vi "Periodic Tasks.vi"(8 "error in (no error)":errorcluster) -> ()   [LabVIEW 2015]
doc: "This VI runs in parallel to other tasks. It can contain as many user-defined periodic loops as you need. These can carry out PID or other sorts of timed response."
uses:
  <vilib>/Rock Robotics/WPI/DriverStation/WPI_DriverStationRobotMode2.ctl
  <vilib>/Rock Robotics/WPI/CAN/TalonSRX/WPI_CANTalonSRX_APIControlMode.ctl
  <vilib>/Rock Robotics/WPI/Utilities/WPI_GetSetVariantRefNum.vi
  Robot Global Data.vi
  <vilib>/Rock Robotics/Network Tables/NT Write Number.vi
  <vilib>/Rock Robotics/Network Tables/NT Write Boolean.vi
  <vilib>/Rock Robotics/Network Tables/SD Read Boolean.vi
  <vilib>/Rock Robotics/Network Tables/SD Write Number.vi
  navX-MXP-LabVIEW/navX-MXP Library/navX-MXP IMU.lvlib
  <vilib>/Rock Robotics/WPI/DriverStation/WPI_DriverStationAllianceInfo.ctl
  900/Team900-VIs/Team900SwerveDrive/Team900SwerveDrive.lvlib
  <vilib>/Rock Robotics/Network Tables/SD Read Number.vi
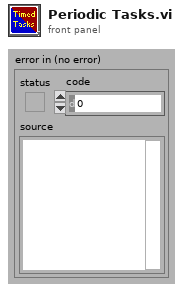
[diagram p1: front panel]
types:
  T1 = typedef "WPI_DriverStationRobotMode2.ctl" = enum16{"Autonomous Disabled", "Autonomous Enabled", "Teleop Disabled", "Teleop Enabled", "Disconnected", "Finish", "Test Disabled", "Test Enabled", "Emergency Stopped"}
  T2 = typedef "WPI_CANTalonSRX_APIControlMode.ctl" = enum8{"Percent VBus", "Speed", "Position", "Slave", "Unchanged / Invalid"}
  T3 = typedef "WPI_MotorControlDeviceRef.ctl" = cluster{"DeviceStatus":errorcluster, "Type":T4, "PWM":cluster{"PWM Channel":T5, "DeadBand":T6}, "CAN":cluster{"Device Number":u8, "Control Mode":T7, "Semaphore":T8, "Max Vout":dbl, "TalonSRX Control Mode":T2}, "Invert":bool, "TransformRef":T9, "InvTransformRef":T9}
  T4 = typedef "WPI_MotorControlType.ctl" = enum16{"PWM", "CAN", "CANTalonSRX"}
  T5 = typedef "FPGA_DIOPWMChannel.ctl" = enum8{"PWM 0", "PWM 1", "PWM 2", "PWM 3", "PWM 4", "PWM 5", "PWM 6", "PWM 7", "PWM 8", "PWM 9", "PWM MXP 0", "PWM MXP 1", "PWM MXP 2", "PWM MXP 3", "PWM MXP 4", "PWM MXP 5", "PWM MXP 6", "PWM MXP 7", "PWM MXP 8", "PWM MXP 9", "Invalid"}
  T6 = typedef "WPI_PWMDeadband.ctl" = cluster{"Name":string, "maxPositivePwm":i32, "minPositivePwm":i32, "centerPwm":i32, "maxNegativePwm":i32, "minNegativePwm":i32, "angularRange":u16}
  T7 = typedef "WPI_CANJaguar_ControlMode.ctl" = enum8{"Percent VBus", "Current", "Speed", "Position", "Voltage"}
  T8 = typedef "Semaphore RefNum" = refnum<k1>
  T9 = typedef "WPI_PWMTransform_ConPane.ctl" = refnum<vi>
  T10 = typedef "WPI_DriverStationAllianceInfo.ctl" = enum16{"Red", "Blue", "Invalid"}
  T11 = cluster{"FL Steering":T3, "FR Steering":T3, "RL Steering":T3, "RR Steering":T3}
  T12 = cluster{"FL Speed":T3, "FR Speed":T3, "RL Speed":T3, "RR Speed":T3}
  T13 = typedef "navX-MXP IMU.lvlib/navX Device TypeDef.ctl" = cluster{"navX Interface Protocol":T14, "navX Interface Protocol TypeDefs":cluster{"SPIDevRef":T15, "I2CDevRef":T17}, "navX System Information":cluster{"Board Information":T19, "Status":T20, "Offsets":T24}, "navX Common Information":cluster{"Update Rate (4Hz-60Hz)":T25, "refnum name":string, "error":errorcluster}}
  T14 = typedef "navX-MXP IMU.lvlib/navX Interface Protocol.ctl" = enum16{"SPI", "I2C"}
  T15 = typedef "WPI_SPIDevRef.ctl" = cluster{"DevStatus":errorcluster, "Handle":i32, "SPI Bus":T16}
  T16 = typedef "spi_bus.ctl" = enum16{"SPI On-Board, CS0", "SPI On-Board, CS1", "SPI On-Board, CS2", "SPI On-Board, CS3", "SPI MXP", "Invalid"}
  T17 = typedef "WPI_I2CDevRef.ctl" = cluster{"DevStatus":errorcluster, "Device Address":u8, "Handle":i32, "I2C Bus":T18}
  T18 = typedef "i2c_bus.ctl" = enum16{"I2C On-Board", "I2C MXP", "Invalid"}
  T19 = typedef "navX-MXP IMU.lvlib/navX Board Information.ctl" = cluster{"WhoAmI (50 | 0x32)":u8, "Board Revision":u8, "Firmware Major Version":u8, "Firmware Minor Version":u8}
  T20 = typedef "navX-MXP IMU.lvlib/navX Status Data.ctl" = cluster{"Update Rate Hz":u8, "Accelerometer Full-Scale Range":u8, "Gyro Full-Scale Range":u16, "NAVX_OP_STATUS":T21, "NAVX_CAL_STATUS":T22, "NAVX_SELFTEST_STATUS":u8, "NAVX_SENSOR_STATUS":T23}
  T21 = typedef "navX-MXP IMU.lvlib/navX NAVX_OP_STATUS.ctl" = u8
  T22 = typedef "navX-MXP IMU.lvlib/navX NAVX_CAL_STATUS.ctl" = u8
  T23 = typedef "navX-MXP IMU.lvlib/navX NAVX_SENSOR_STATUS.ctl" = cluster{"MOVING":bool, "YAW_STABLE":bool, "MAG_DISTURBANCE":bool, "ALTITUDE_VALID":bool, "SEALEVEL_PRESS_SET":bool, "FUSED_HEADING_VALID":bool}
  T24 = typedef "navX-MXP IMU.lvlib/navX Offsets Data.ctl" = cluster{"Yaw":dbl, "Quat W":dbl, "Quat X":dbl, "Quat Y":dbl, "Quat Z":dbl}
  T25 = typedef "navX-MXP IMU.lvlib/navX Update Rate.ctl" = u8
  T26 = typedef "navX-MXP IMU.lvlib/navX YPRH Data.ctl" = cluster{"Yaw":dbl, "Pitch":dbl, "Roll":dbl, "Heading":dbl}
  T27 = typedef "WPI_CANTalonSRX_GlobalStatus.ctl" = cluster{"Applied Throttle":dbl, "Module Enabled":bool, "CAN Error":errorcluster, "Closed Loop Error":dbl, "Forward Limit Switch Closed":bool, "Reverse Limit Switch Closed":bool, "Sensor Position":dbl, "Sensor Velocity":dbl, "Current":dbl, "Sticky Fault - Over Temp":bool, "Sticky Fault - Under Voltage":bool, "Sticky Fault - Forward Limit":bool, "Sticky Fault - Reverse Limit":bool, "Sticky Fault - Forward Soft Limit":bool, "Sticky Fault - Reverse Soft Limit":bool, "Brake is Enabled":bool, "Encoder Position":dbl, "Encoder Velocity":dbl, "Encoder Index Count":dbl, "Encoder A Pin State":bool, "Encoder B Pin State":bool, "Encoder Index Pin State":bool, "Analog In":dbl, "Analog In Velocity":dbl, "Temperature (C)":dbl, "Battery Voltage":dbl}
  T28 = cluster{"[0]":dbl, "[1]":dbl, "[2]":dbl, "[3]":dbl}
  T29 = typedef "WPI_DriverStationPositionInfo.ctl" = enum16{"1", "2", "3"}
  T30 = typedef "WPI_JoystickDevRef.ctl" = cluster{"Device":T31}
  T31 = typedef "WPI_JoystickDeviceEnum.ctl" = enum16{"USB 0", "USB 1", "USB 2", "USB 3", "USB 4", "USB 5"}
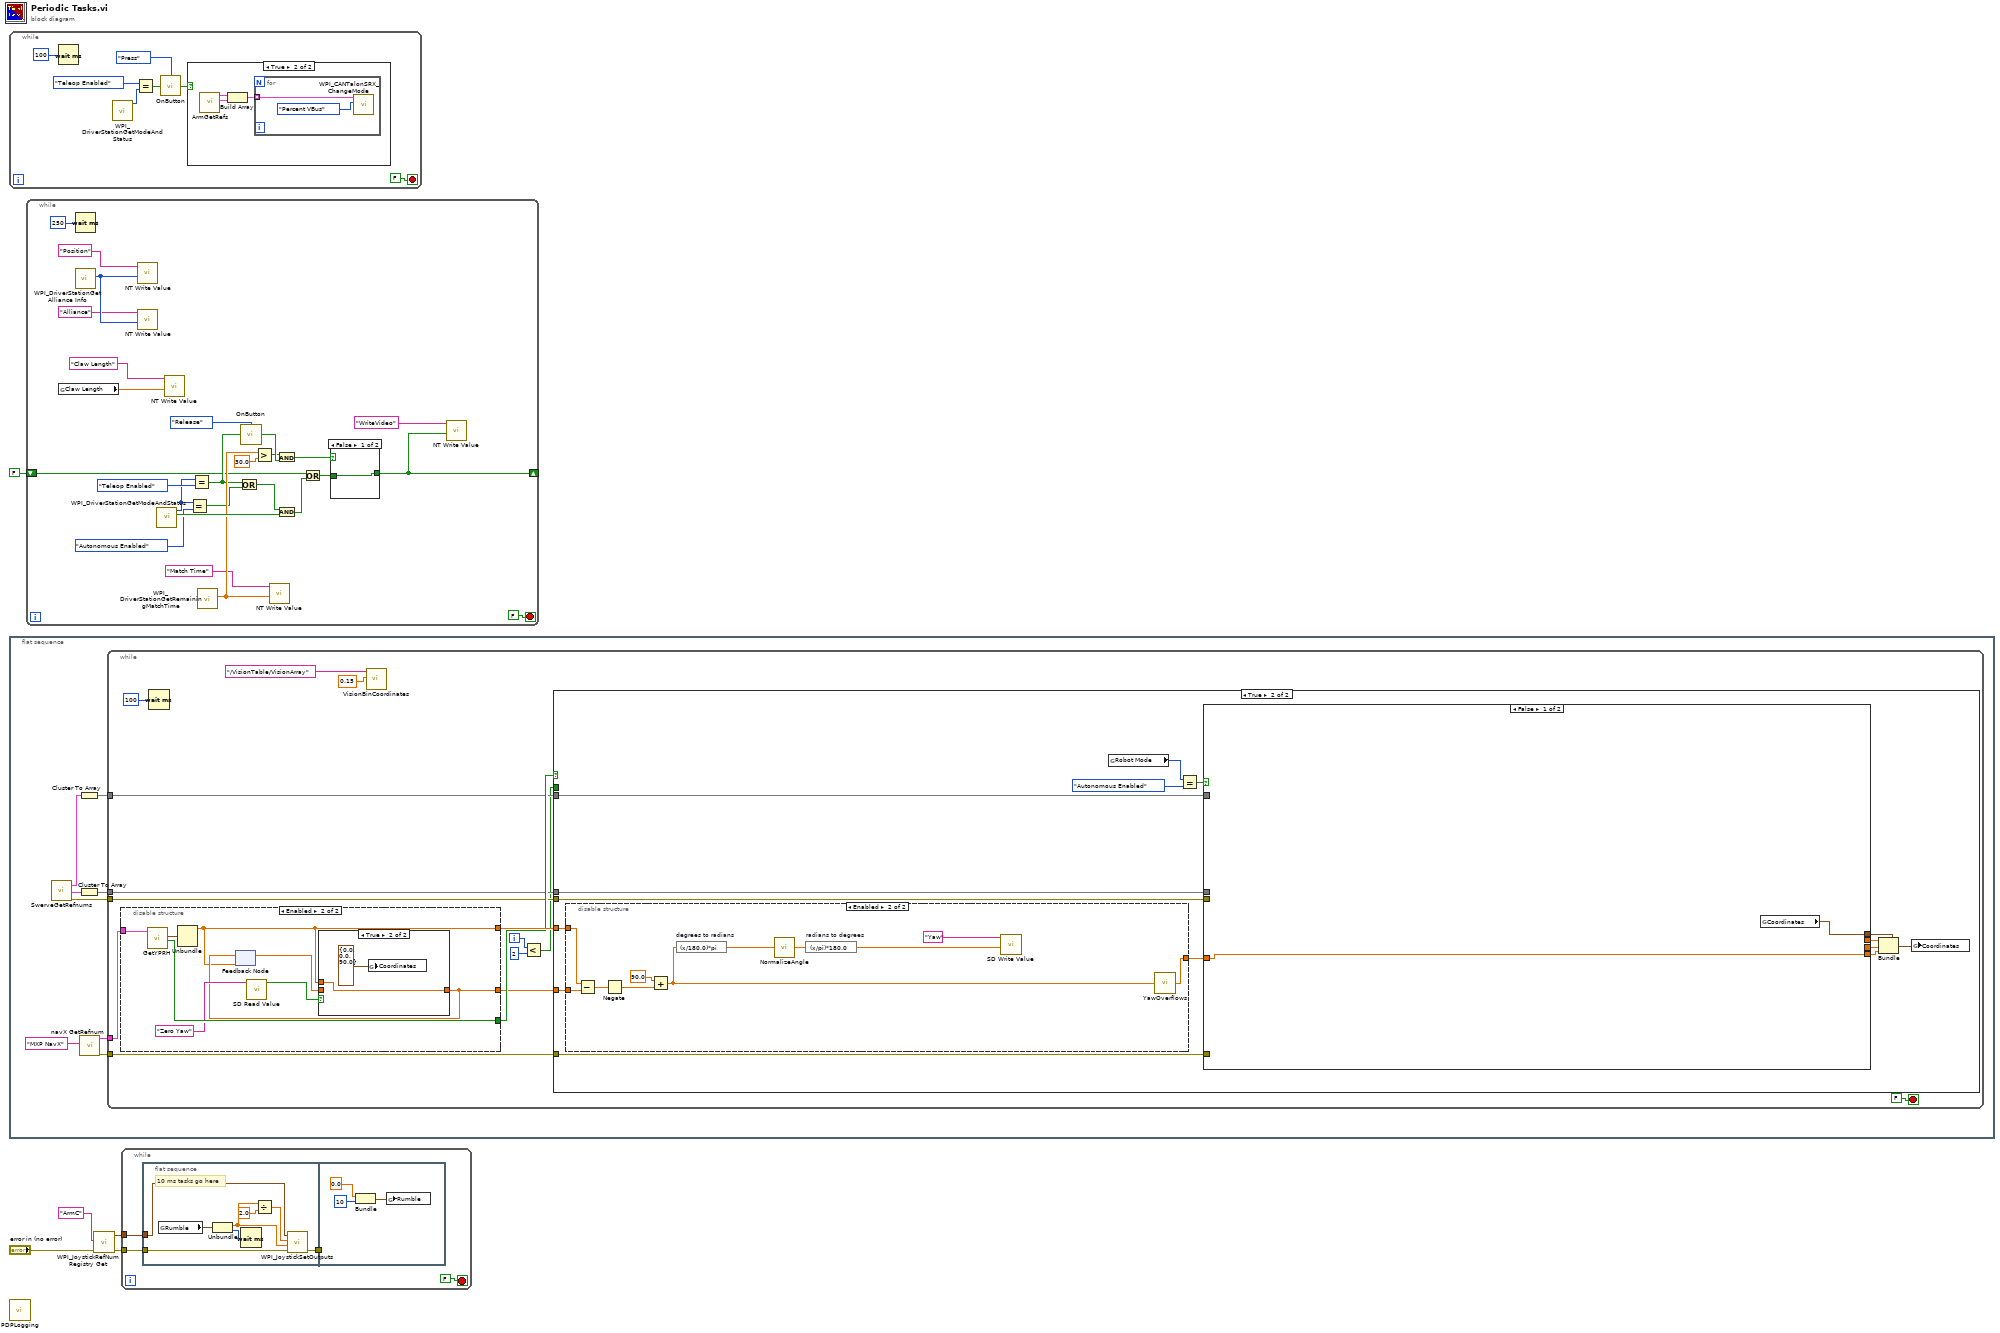
[diagram p0: block diagram]
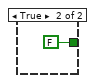
[diagram p3: hidden frame]
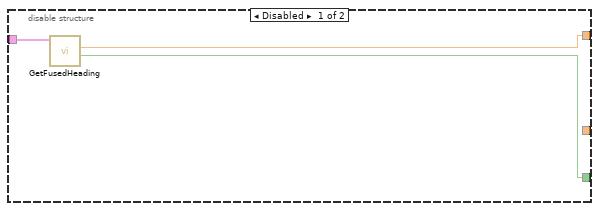
[diagram p4: hidden frame]
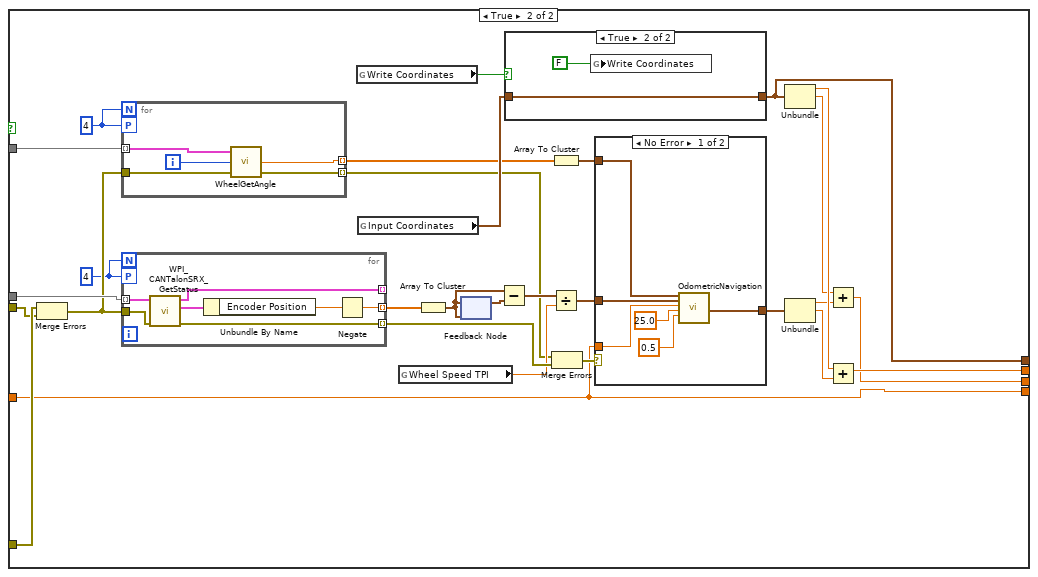
[diagram p7: hidden frame]
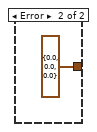
[diagram p8: hidden frame]
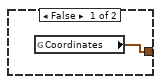
[diagram p9: hidden frame]
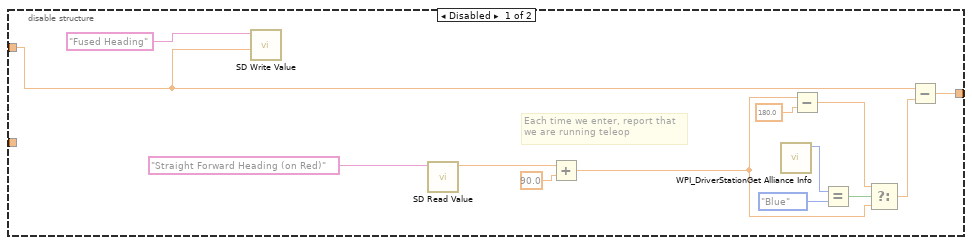
[diagram p10: hidden frame]
diagram:
  n1 = while {
    stop <- FALSE stop-if-true
    n2 = Wait (ms)(milliseconds to wait=u32 100) -> ()  [unwired: 1 out]
    n3 = call <vilib>:"WPI_DriverStationGetModeAndStatus.vi"() -> ("Robot Mode"=w9:T1)  [unwired: 10 in, 1 out]
    n4 = Equal?(x=WPI_DriverStationRobotMode2."Teleop Enabled" ("Robot Mode"), y=w9) -> (x = y?=w8:bool)
    n5 = call "OnButton.vi"("Button"=w8, "Mode"=enum16{"Press", "Release", "Both"}."Press") -> ("Value"=w11:bool)
    n6 = case shown="True" w11 {
      frame False {
      }
      frame True {
        n7 = call "ArmGetRefs.vi"() -> ("Extension Ref"=w15:T3, "Pivot Ref"=w14:T3)  [unwired: 8 in, 2 out]
        n8 = Build Array(w14, w15) -> (w13:T3[])
        n9 = for {
          tunnel: w13 -> [w17] mode=indexing
          n10 = call <vilib>:"WPI_CANTalonSRX_ChangeMode.vi"("Control Mode"=WPI_CANTalonSRX_APIControlMode."Percent VBus", "CAN Talon SRX Ref"=w17) -> ()  [unwired: 8 in, 2 out]
        }
      }
    }
  }
  n11 = flat-sequence {
    frame #0 {
      n12 = call "SwerveGetRefnums.vi"() -> ("Steering"=w19:T11, "Speed"=w21:T12, "error out"=w20:errorcluster)  [unwired: 9 in, 8 out]
      n13 = Cluster To Array(cluster=w19) -> (array=w18:T3[])
      n14 = Cluster To Array(cluster=w21) -> (array=w22:T3[])
      n15 = call "navX GetRefnum.vi"("refnum name"="MXP NavX") -> ("error out"=w23:errorcluster, "navX Device TypeDef"=w24:T13)  [unwired: 9 in]
      n16 = while {
        tunnel: w24 -> [w37]
        tunnel: w23 -> [w36]
        tunnel: w20 -> [w32]
        tunnel: w22 -> [w33]
        tunnel: w18 -> [w31]
        i -> [w30]
        stop <- FALSE stop-if-true
        n17 = disable-structure shown="Enabled" {
          disable-tunnel: [w43 w44] -> w39
          disable-tunnel: [w42 w49] -> w38
          disable-tunnel: w37 -> [w41 w51]
          disable-tunnel: [_ w46] -> w35
          frame Disabled {
            n18 = call "GetFusedHeading.vi"("navX Device TypeDef"=w41) -> ("Valid?"=w42:bool, "Fused Heading"=w43:dbl)  [unwired: 8 in, 1 out]
          }
          frame Enabled {
            n19 = call "GetYPRH.vi"("navX Device TypeDef"=w51) -> ("Valid?"=w49:bool, "YPRH"=w50:T26)  [unwired: 8 in, 1 out]
            n20 = Unbundle(w50) -> ("Yaw"=w44:dbl)  [unwired: 3 out]
            n21 = feedback #1(w44) -> (w47:dbl)
            n22 = call-poly <vilib>:"SD Read Value.vi"("Name"="Zero Yaw") -> ("Boolean"=w45:bool)  [unwired: 8 in, 2 out]
            n23 = case shown="True" w45 {
              tunnel: w44 -> [_ w54]
              tunnel: [w52 w54] -> w46
              tunnel: w47 -> [w52 _]
              frame False {
              }
              frame True {
                n24 = global write "Robot Global Data.vi" "Coordinates"(cluster{"X":dbl, "Y":dbl, "Heading":dbl} {"X"=0.0, "Y"=0.0, "Heading"=90.0} ("Coordinates")) -> ()
              }
            }
            n25 = feedback-in #1(w46) -> ()
          }
        }
        n26 = Wait (ms)(milliseconds to wait=u32 100) -> ()  [unwired: 1 out]
        n27 = call "VisionBinCoordinates.vi"("Minimum Ratio"=0.15, "Vision Array Name"="/VisionTable/VisionArray") -> ()  [unwired: 2 in, 5 out]
        n28 = Less?(x=w30, y=2) -> (x < y?=w28:bool)
        n29 = case shown="True" w38 {
          tunnel: w39 -> [_ w69]
          tunnel: w36 -> [_ w68]
          tunnel: w35 -> [_ w67]
          tunnel: w33 -> [_ w66]
          tunnel: w32 -> [_ w65]
          tunnel: w31 -> [_ w64]
          tunnel: w28 -> [_ _]
          frame False {
          }
          frame True {
            n30 = disable-structure shown="Enabled" {
              disable-tunnel: [w134 w137] -> w63
              disable-tunnel: w69 -> [w133 w145]
              disable-tunnel: w67 -> [_ w144]
              frame Disabled {
                # "Each time we enter, report that\nwe are running teleop"
                n31 = call-poly <vilib>:"SD Write Value.vi"("Numeric"=w133, "Name"="Fused Heading") -> ()  [unwired: 8 in, 2 out]
                n32 = call-poly <vilib>:"SD Read Value.vi"("Name"="Straight Forward Heading (on Red)") -> ("Numeric"=w126:dbl)  [unwired: 8 in, 2 out]
                n33 = Add(x=w126, y=90.0) -> (x+y=w124:dbl)
                n34 = call <vilib>:"WPI_DriverStationGet Alliance Info.vi"() -> ("Alliance"=w130:T10)  [unwired: 10 in, 1 out]
                n35 = Subtract(x=w124, y=180.0) -> (x-y=w127:dbl)
                n36 = Equal?(x=w130, y=WPI_DriverStationAllianceInfo."Blue") -> (x = y?=w128:bool)
                n37 = Select(t=w127, s=w128, f=w124) -> (s? t:f=w135:dbl)
                n38 = Subtract(x=w133, y=w135) -> (x-y=w134:dbl)
              }
              frame Enabled {
                n39 = Subtract(x=w145, y=w144) -> (x-y=w142:dbl)
                n40 = Negate(x=w142) -> (-x=w143:dbl)
                n41 = Add(x=90.0, y=w143) -> (x+y=w138:dbl)
                n42 = expression code="(x/180.0)*pi" "degrees to radians"(w138) -> (w139:dbl)
                n43 = call "NormalizeAngle.vi"("angle (rad)"=w139) -> ("angle (between pi and -pi)"=w136:dbl)
                n44 = expression code="(x/pi)*180.0" "radians to degrees"(w136) -> (w140:dbl)
                n45 = call-poly <vilib>:"SD Write Value.vi"("Numeric"=w140, "Name"="Yaw") -> ()  [unwired: 8 in, 2 out]
                n46 = call "YawOverflows.vi"("Yaw (degrees)"=w138) -> ("Yaw (with overflows)"=w137:dbl)
              }
            }
            n47 = global read "Robot Global Data.vi" "Robot Mode"() -> (w62:T1)
            n48 = Equal?(x=w62, y=WPI_DriverStationRobotMode2."Autonomous Enabled") -> (x = y?=w60:bool)
            n49 = case shown="False" w60 {
              tunnel: w68 -> [_ w96]
              tunnel: w66 -> [_ w95]
              tunnel: w65 -> [_ w94]
              tunnel: w64 -> [_ w93]
              tunnel: w63 -> [w71 w72]
              tunnel: [w70 w75] -> w58
              tunnel: [_ w74] -> w57
              tunnel: [_ w73] -> w56
              tunnel: [w71 w72] -> w55
              frame False {
                n50 = global read "Robot Global Data.vi" "Coordinates"() -> (w70:cluster{"X":dbl, "Y":dbl, "Heading":dbl})
              }
              frame True {
                w76 = 4
                w77 = 4
                n51 = Merge Errors(w96, w94) -> (w81:errorcluster)
                n52 = for {
                  N: w76 -> [_]
                  workers-P: w76 -> [_]
                  tunnel: w81 -> [w104]
                  tunnel: [w103] -> w80 mode=indexing
                  tunnel: w93 -> [w102] mode=indexing
                  tunnel: [w101] -> w78 mode=indexing
                  i -> [w105]
                  n53 = call "WheelGetAngle.vi"("error in (no error)"=w104, "Wheel"=w105, "CAN Talon SRX Ref"=w102) -> ("error out"=w103:errorcluster, "Sensor Position (rad)"=w101:dbl)  [unwired: 1 out]
                }
                n54 = for {
                  N: w77 -> [_]
                  tunnel: [w117] -> _ mode=indexing
                  tunnel: [w119] -> w89 mode=indexing
                  workers-P: w77 -> [_]
                  tunnel: w95 -> [w116] mode=indexing
                  tunnel: [w114] -> w83 mode=indexing
                  tunnel: w81 -> [w115]
                  n55 = call <vilib>:"WPI_CANTalonSRX_GetStatus.vi"("error in (no error)"=w115, "CAN Talon SRX Ref"=w116) -> ("error out"=w119:errorcluster, "Talon SRX Status"=w118:T27, "CAN Talon SRX Ref"=w117:T3)  [unwired: 7 in]
                  n56 = Unbundle By Name(w118) -> ("Encoder Position"=w113:dbl)
                  n57 = Negate(x=w113) -> (-x=w114:dbl)
                }
                n58 = global read "Robot Global Data.vi" "Write Coordinates"() -> (w91:bool)
                n59 = global read "Robot Global Data.vi" "Input Coordinates"() -> (w92:cluster{"X":dbl, "Y":dbl, "Heading":dbl})
                n60 = global read "Robot Global Data.vi" "Wheel Speed TPI"() -> (w82:dbl)
                n61 = Array To Cluster(array=w83) -> (cluster=w84:T28)
                n62 = feedback #2(w84) -> (w85:T28)
                n63 = feedback-in #2(w84) -> ()
                n64 = Subtract(x=w84, y=w85) -> (x-y=w86:T28)
                n65 = case shown="True" w91 {
                  tunnel: [w120 w122] -> w75
                  tunnel: w92 -> [_ w122]
                  frame False {
                    n66 = global read "Robot Global Data.vi" "Coordinates"() -> (w120:cluster{"X":dbl, "Y":dbl, "Heading":dbl})
                  }
                  frame True {
                    n67 = global write "Robot Global Data.vi" "Write Coordinates"(FALSE) -> ()
                  }
                }
                n68 = Array To Cluster(array=w78) -> (cluster=w79:T28)
                n69 = Divide(x=w86, y=w82) -> (x/y=w87:T28)
                n70 = Merge Errors(w80, w89) -> (w88:errorcluster)
                n71 = case shown="No Error" w88 {
                  tunnel: [w109 cluster{"sy":dbl, "sx":dbl, "rot.":dbl} {"sy"=0.0, "sx"=0.0, "rot."=0.0} ("movement")] -> w90
                  tunnel: w87 -> [w111 _]
                  tunnel: w79 -> [w110 _]
                  tunnel: w72 -> [w106 _]
                  frame No Error {
                    n72 = call "OdometricNavigation.vi"("Wheel Angles (rad)"=w110, "Wheel Movements (in.)"=w111, "Robot angle (degrees)"=w106, "x and y error minimum (in.)"=25.0, "error minimum for rotation (rad)"=0.5 ("error minimum for rotation (in.)")) -> ("movement"=w109:cluster{"sy":dbl, "sx":dbl, "rot.":dbl})  [unwired: 14 in]
                  }
                  frame Error {
                  }
                }
                n73 = Unbundle(w75) -> ("X"=w100:dbl, "Y"=w98:dbl)  [unwired: 1 out]
                n74 = Unbundle(w90) -> ("sy"=w97:dbl, "sx"=w99:dbl)  [unwired: 1 out]
                n75 = Add(x=w98, y=w97) -> (x+y=w73:dbl)
                n76 = Add(x=w100, y=w99) -> (x+y=w74:dbl)
              }
            }
            n77 = Bundle(cluster=w58, "X"=w57, "Y"=w56, "Heading"=w55) -> (w59:cluster{"X":dbl, "Y":dbl, "Heading":dbl})
            n78 = global write "Robot Global Data.vi" "Coordinates"(w59) -> ()
          }
        }
      }
    }
  }
  n79 = call "PDPLogging.vi"() -> ()  [unwired: 12 in]
  n80 = while {
    shift-right: [w151] -> _
    shift-left: FALSE -> [w152]
    stop <- FALSE stop-if-true
    n81 = global read "Robot Global Data.vi" "Claw Length"() -> (w149:dbl)
    n82 = call <vilib>:"WPI_DriverStationGet Alliance Info.vi"() -> ("Position"=w148:T29)  [unwired: 10 in, 1 out]
    n83 = Wait (ms)(milliseconds to wait=250) -> ()  [unwired: 1 out]
    n84 = call-poly <vilib>:"NT Write Value.vi"("Numeric"=w148, "Name"="Position") -> ()  [unwired: 9 in, 1 out]
    n85 = call-poly <vilib>:"NT Write Value.vi"("Numeric"=w148, "Name"="Alliance") -> ()  [unwired: 9 in, 1 out]
    n86 = call <vilib>:"WPI_DriverStationGetModeAndStatus.vi"() -> ("FMS Attached"=w170:bool, "Robot Mode"=w157:T1)  [unwired: 10 in]
    n87 = call-poly <vilib>:"NT Write Value.vi"("Numeric"=w149, "Name"="Claw Length") -> ()  [unwired: 9 in, 1 out]
    n88 = Equal?(x=w157, y=WPI_DriverStationRobotMode2."Autonomous Enabled") -> (x = y?=w154:bool)
    n89 = Equal?(x=w157, y=WPI_DriverStationRobotMode2."Teleop Enabled" ("Robot Mode")) -> (x = y?=w153:bool)
    n90 = call <vilib>:"WPI_DriverStationGetRemainingMatchTime.vi"() -> ("Match Time(s)"=w160:sgl)  [unwired: 10 in, 1 out]
    n91 = Or(x=w153, y=w154) -> (x .or. y?=w155:bool)
    n92 = call "OnButton.vi"("Button"=w153, "Mode"=enum16{"Press", "Release", "Both"}."Release") -> ("Value"=w165:bool)
    n93 = Greater?(x=w160, y=sgl 30.0) -> (0:w162:bool)
    n94 = call-poly <vilib>:"NT Write Value.vi"("Numeric"=w160, "Name"="Match Time") -> ()  [unwired: 9 in, 1 out]
    n95 = And(x=w162, y=w165) -> (x .and. y?=w163:bool)
    n96 = And(x=w155, y=w170) -> (x .and. y?=w166:bool)
    n97 = Or(x=w152, y=w166) -> (x .or. y?=w167:bool)
    n98 = case shown="False" w163 {
      tunnel: [w173 FALSE] -> w151
      tunnel: w167 -> [w173 _]
      frame False {
      }
      frame True {
      }
    }
    n99 = call-poly <vilib>:"NT Write Value.vi"("Boolean"=w151, "Name"="WriteVideo") -> ()  [unwired: 9 in, 1 out]
  }
  n100 = call <vilib>:"WPI_JoystickRefNum Registry Get.vi"("error in (no error)"="error in (no error)", "refnum name"="ArmC") -> ("error out"=w4:errorcluster, "JoystickDevRef"=w2:T30)  [unwired: 8 in]
  n101 = while {
    tunnel: w4 -> [w177]
    tunnel: w2 -> [w176]
    stop <- FALSE stop-if-true
    n102 = flat-sequence {
      tunnel: w177 -> [w184]
      tunnel: w176 -> [w183]
      tunnel: [w179] -> w175
      tunnel: w175 -> [_]
      frame #0 {
        # "10 ms tasks go here"
        n103 = global read "Robot Global Data.vi" "Rumble"() -> (w182:cluster{"Intensity":dbl, "Duration":i16})
        n104 = Unbundle(w182) -> ("Intensity"=w181:dbl, "Duration"=w180:i16)
        n105 = Wait (ms)(milliseconds to wait=w180) -> ()  [unwired: 1 out]
        n106 = Divide(x=w181, y=2.0) -> (x/y=w185:dbl)
        n107 = call <vilib>:"WPI_JoystickSetOutputs.vi"("error in (no error)"=w184, "Right Rumble"=w181, "Left Rumble"=w185, "JoystickDevRef"=w183) -> ("error out"=w179:errorcluster)  [unwired: 6 in, 1 out]
      }
      frame #1 {
        n108 = Bundle("t"=0.0, "f"=i16 10) -> (w187:cluster{"t":dbl, "f":i16})  [unwired: 1 in]
        n109 = global write "Robot Global Data.vi" "Rumble"(w187) -> ()
      }
    }
  }
